vi "TrashCan.vi"() -> ()   [LabVIEW 2020]
panel:
  out "Trash Can":dbl(slide) scale=0.0..500.0
  out "Lid Status":string
  out "Clean Trash":bool
  out "Sonar Reading [Available Space]":dbl(graph)
  out "Space Available":bool
  in  "Table Control":string[][](table)
  in  "VISA resource name":refnum<visa-resource-name>
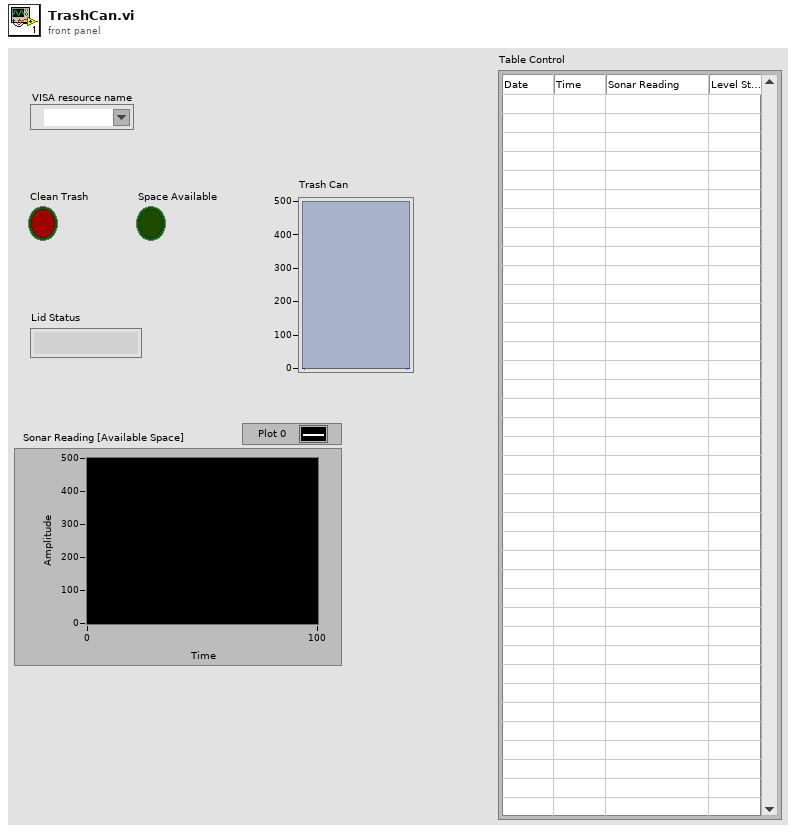
[diagram p1: front panel]
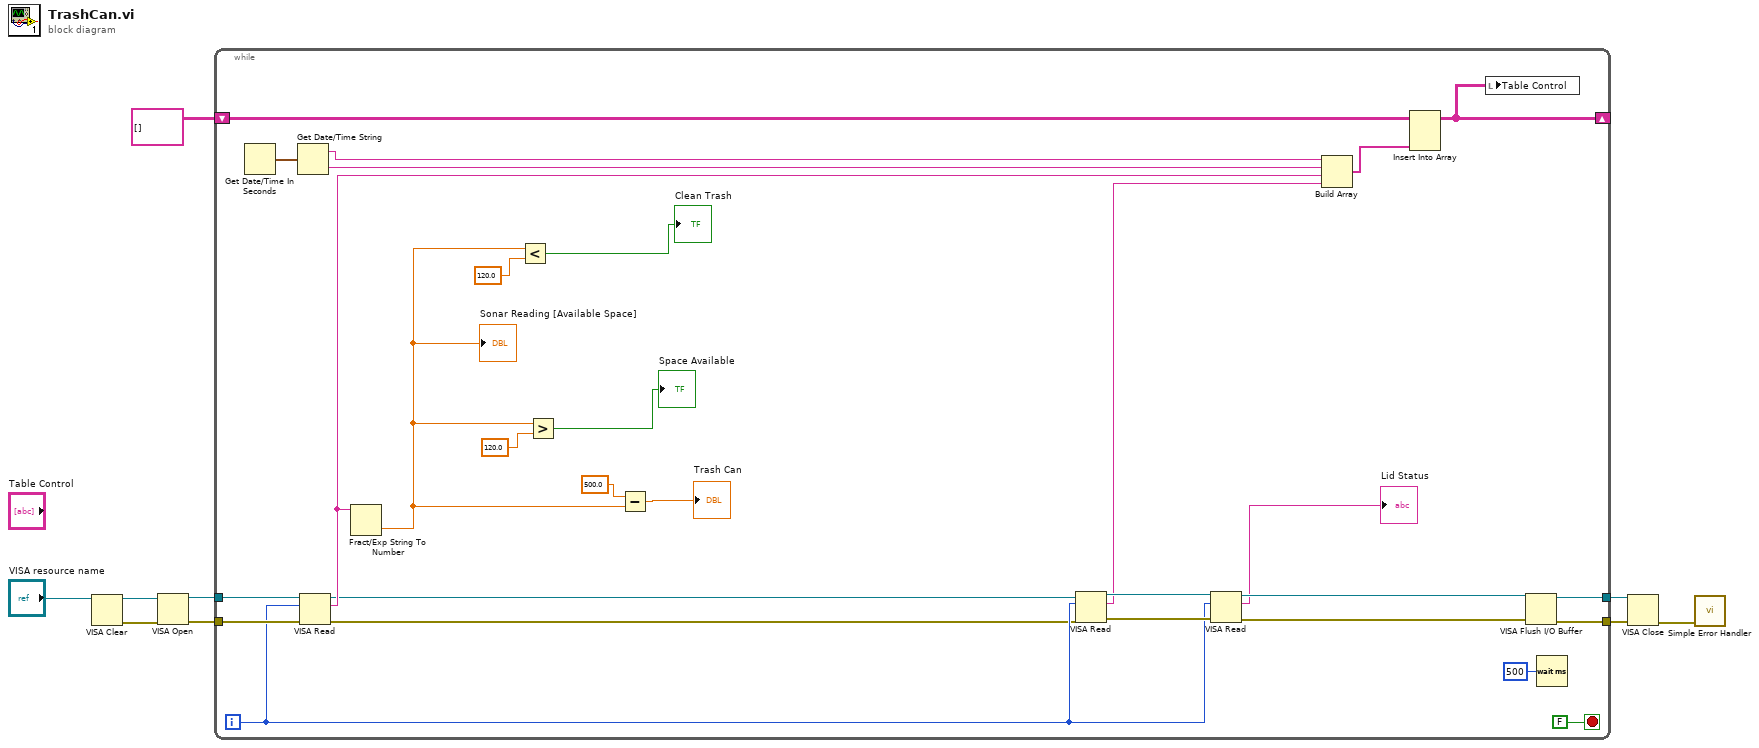
[diagram p0: block diagram]
diagram:
  n1 = VISA Clear(VISA resource name="VISA resource name") -> (VISA resource name out=w7:refnum<visa-resource-name>, error out=w6:errorcluster)  [unwired: 1 in]
  n2 = VISA Open(error in (no error)=w6, VISA resource name=w7) -> (VISA resource name=w9:refnum<visa-resource-name>, error out=w8:errorcluster)  [unwired: 3 in]
  n3 = while {
    tunnel: w9 -> [w38]
    tunnel: w8 -> [w37]
    tunnel: [w36] -> w5
    tunnel: [w35] -> w4
    shift-right: [w31] -> _
    shift-left: string[][] [] -> [w32]
    i -> [w19]
    stop <- FALSE stop-if-true
    n4 = Get Date/Time In Seconds() -> (seconds since 1Jan1904=w30:timestamp)
    n5 = Get Date/Time String(seconds (now)=w30) -> (date string=w10:string, time string=w29:string)  [unwired: 2 in]
    n6 = VISA Read(VISA resource name=w38, byte count=w19, error in (no error)=w37) -> (VISA resource name out=w16:refnum<visa-resource-name>, read buffer=w27:string, error out=w15:errorcluster)  [unwired: 1 out]
    n7 = Fract/Exp String To Number(string=w27) -> (number=w13:dbl)  [unwired: 3 in, 1 out]
    "Sonar Reading [Available Space]" <- w13
    n8 = Less?(x=w13, y=120.0) -> (x < y?=→"Clean Trash":bool)
    n9 = Greater?(x=w13, y=120.0) -> (0:→"Space Available":bool)
    n10 = Subtract(x=500.0, y=w13) -> (x-y=→"Trash Can":dbl)
    n11 = VISA Read(VISA resource name=w16, byte count=w19, error in (no error)=w15) -> (VISA resource name out=w24:refnum<visa-resource-name>, read buffer=w22:string, error out=w23:errorcluster)  [unwired: 1 out]
    n12 = VISA Read(VISA resource name=w24, byte count=w19, error in (no error)=w23) -> (VISA resource name out=w21:refnum<visa-resource-name>, read buffer=→"Lid Status":string, error out=w20:errorcluster)  [unwired: 1 out]
    n13 = Build Array(w10, w29, w27, w22) -> (w28:string[])
    n14 = Insert Into Array(array=w32, new element=w28) -> (w31:string[][])  [unwired: 2 in]
    n15 = local write "Table Control"(w31) -> ()
    n16 = VISA Flush I/O Buffer(VISA resource name=w21, error in (no error)=w20) -> (VISA resource name out=w36:refnum<visa-resource-name>, error out=w35:errorcluster)  [unwired: 1 in]
    n17 = Wait (ms)(milliseconds to wait=u32 500) -> ()  [unwired: 1 out]
  }
  n18 = VISA Close(VISA resource name=w5, error in (no error)=w4) -> (error out=w3:errorcluster)
  n19 = call <vilib>:"Simple Error Handler.vi"("error in (no error)"=w3) -> ()  [unwired: 4 in, 5 out]
